vi "20220401.SA40289B 1D+2D in Air Dec.vi"() -> ()   [LabVIEW 2019]
uses:
  <userlib>/LevyLab/XY Utilities/subVIs/Get X and Y (multiple).vi
  <vilib>/Analysis/baseanly.llb/Mean (DBL).vi
  <userlib>/LevyLab/XY Utilities/subVIs/Linear Fit (single).vi
  <userlib>/LevyLab/XY Utilities/subVIs/Get X and Y (single).vi
  <userlib>/LevyLab/XY Utilities/Swap X and Y.vi
  <userlib>/LevyLab/XY Utilities/subVIs/Swap X and Y (single).vi
  <vilib>/Analysis/6fits.llb/Linear Fit Intervals.vi
  <vilib>/Analysis/6fits.llb/Confidence Interval (Linear).vi
  <userlib>/_OpenG.lib/file/file.llb/Build Path - Traditional__ogtk.vi
  <userlib>/LevyLab/XY Utilities/XY to 2D.vi
  <userlib>/LevyLab/Control VI/Other/Ramp_SubVI.vi
  <userlib>/LevyLab/LV-Data/LV-Data/LV-Data.lvclass
  <userlib>/LevyLab/XY Utilities/xy_utilities.lvlib
  <vilib>/Analysis/NI_AALBase.lvlib
panel:
  out "E_a":dbl[](array[numeric])
  out "Increasing Temp?":bool=TRUE
  out "Environment":enum16{"Air/Helium", "Vacuum"}(ring)
  in  "Tab Control":enum32{"Page 1", "Page 2"}(tab)
  out "G2T":cluster{dbl[], dbl[]}[](graph)
  out "Temp":cluster{dbl[], dbl[]}[](graph)
  out "Slopes vs Temp":cluster{dbl[], dbl[]}[](graph)
  out "Arrhenius":cluster{dbl[], dbl[]}[](graph)
  out "G4T 2D":cluster{dbl[], dbl[]}[](graph)
  out "G4T 1D":cluster{dbl[], dbl[]}[](graph)
  out "Temp 2":cluster{dbl[], dbl[]}[](graph)
  in  "Arrhenius?":bool=TRUE
  in  "2D Data?":bool=TRUE
  in  "Source Voltage":dbl=0.1
  in  "Init Temp":i32=275
  in  "Temp Step":i32=5
  in  "Final Temp":i32=300
  in  "Trimming":i32=400
  in  "Path":path=path "G:/.shortcut-targets-by-id/0B8-gGFa6hkR4XzJJMDlqZXVKRk0/ansom/Data/PPMS 2/SA40289B.20220401/00 - test/SA40289B.20220401.275K.dat"
  in  "One File?":bool
  in  "OK":bool
  in  "Update":bool
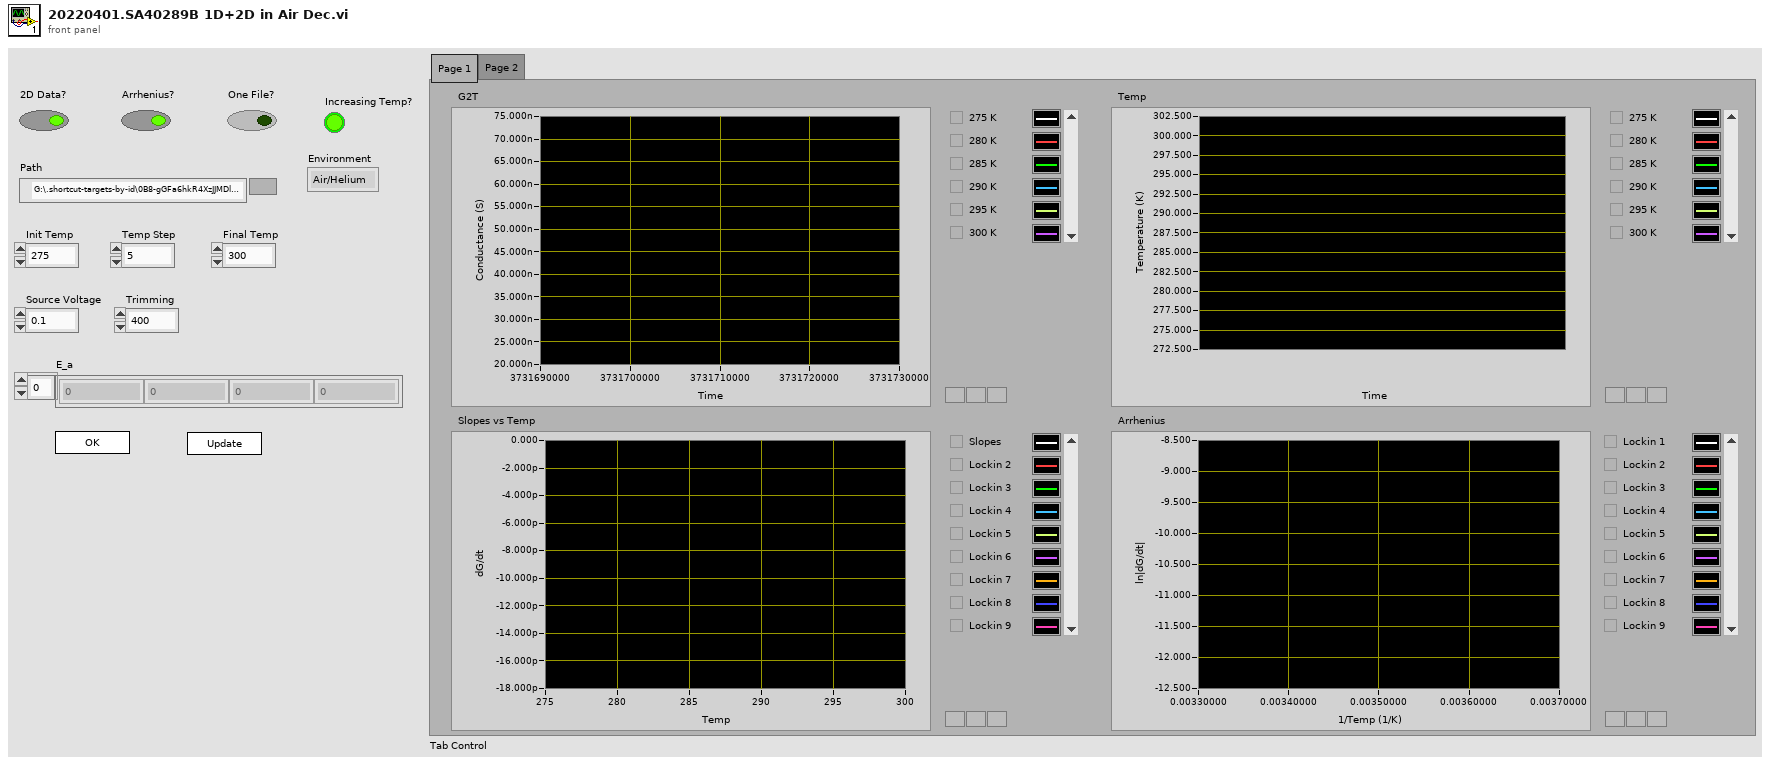
[diagram p1: front panel]
types:
  T1 = enum32{"Invalid", "Standard", "Closed", "Hidden", "Minimized", "Maximized"}
  T2 = enum32{"invalid app kind", "Development System", "Run Time System", "Student Edition", "Embedded LabVIEW", "Evaluation", "Custom"}
  T3 = cluster{"Core":cluster{"Current VI Reference":refnum<vi>, "Close Panel on Exit?":bool}, "G2T":cluster{dbl[], dbl[]}[], "G4T 1D":cluster{dbl[], dbl[]}[], "G4T 2D":cluster{dbl[], dbl[]}[], "Temp":cluster{dbl[], dbl[]}[], "Slopes":cluster{dbl[], dbl[]}[], "Source Voltage":dbl, "Final Temp":i32, "Init Temp":i32, "Temp Step":i32, "Trimming":i32, "Path":path, "One File?":bool}
  T4 = cluster{"Current VI Reference":refnum<vi>, "Close Panel on Exit?":bool}
  T5 = typedef "LV-Data.lvclass/Dictionary--cluster.ctl" = cluster{"key":string, "value":variant}
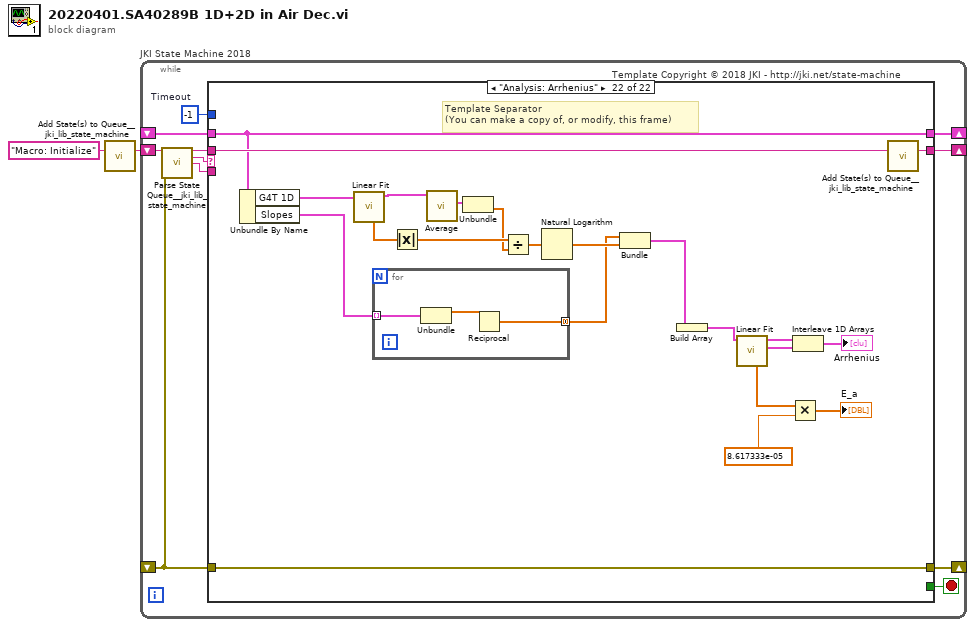
[diagram p0: block diagram]
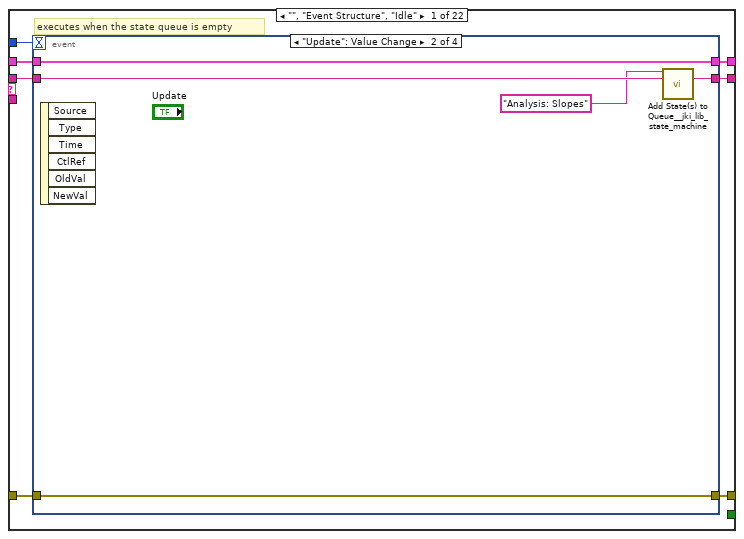
[diagram p2: hidden frame]
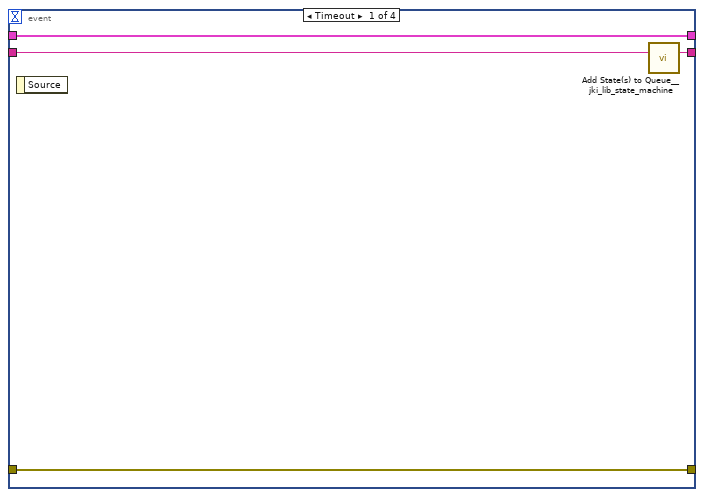
[diagram p3: hidden frame]
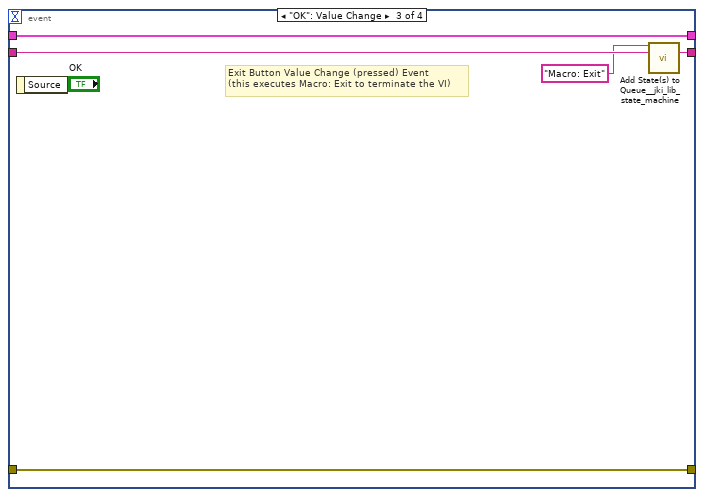
[diagram p4: hidden frame]
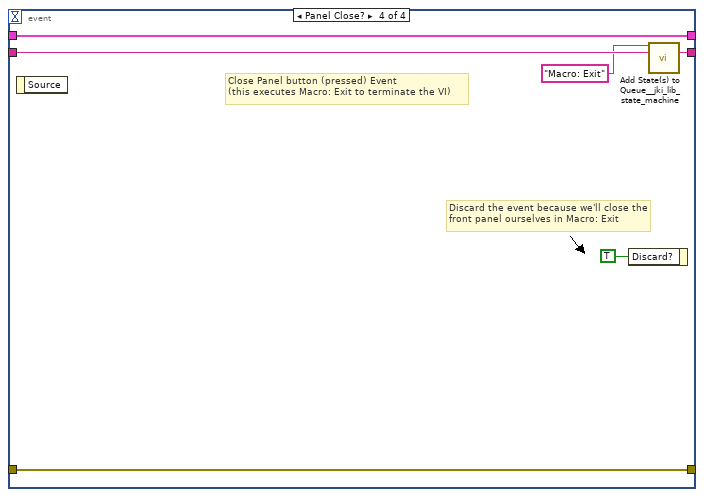
[diagram p5: hidden frame]
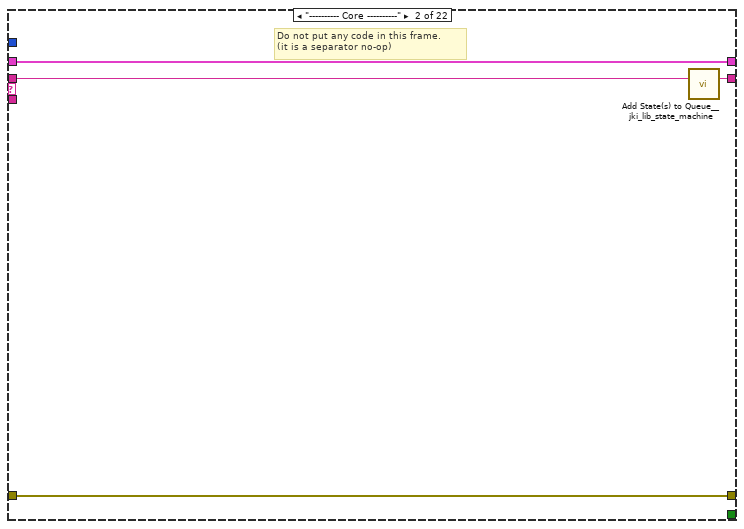
[diagram p6: hidden frame]
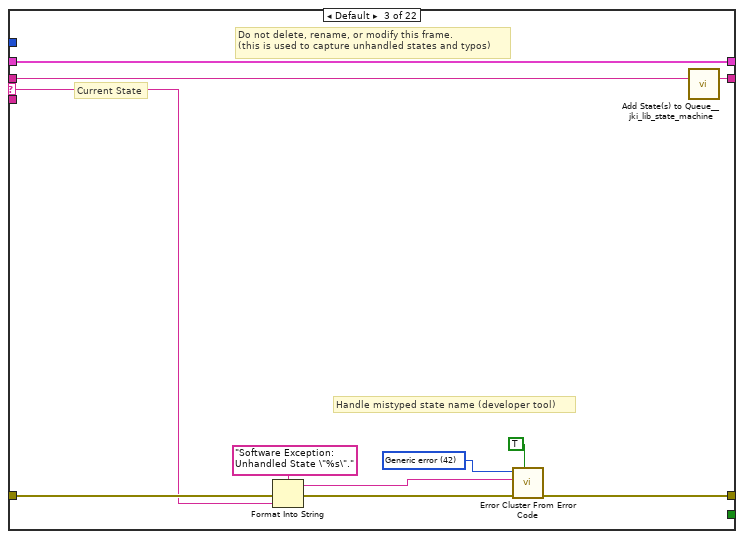
[diagram p7: hidden frame]
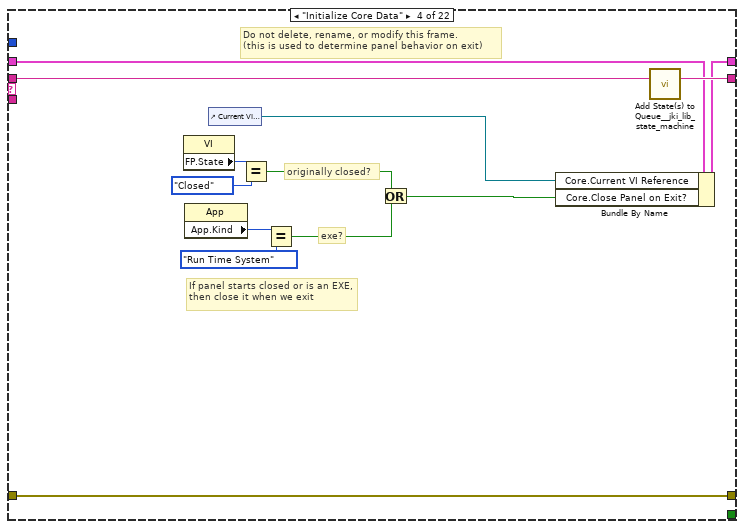
[diagram p8: hidden frame]
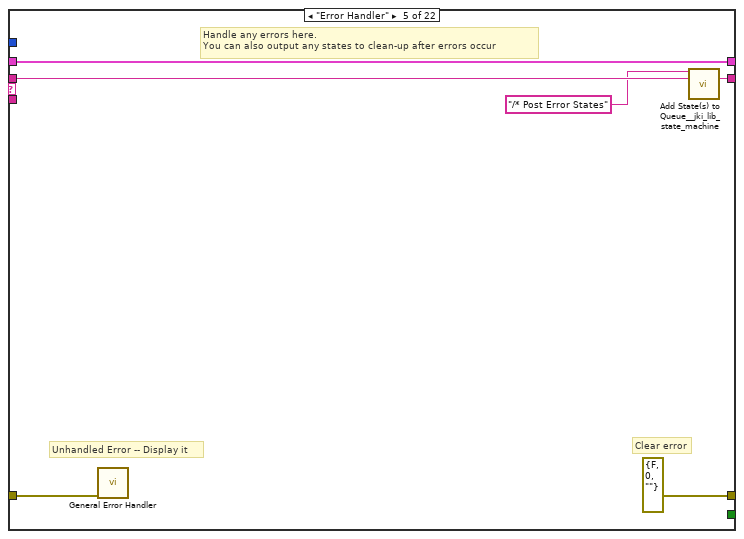
[diagram p9: hidden frame]
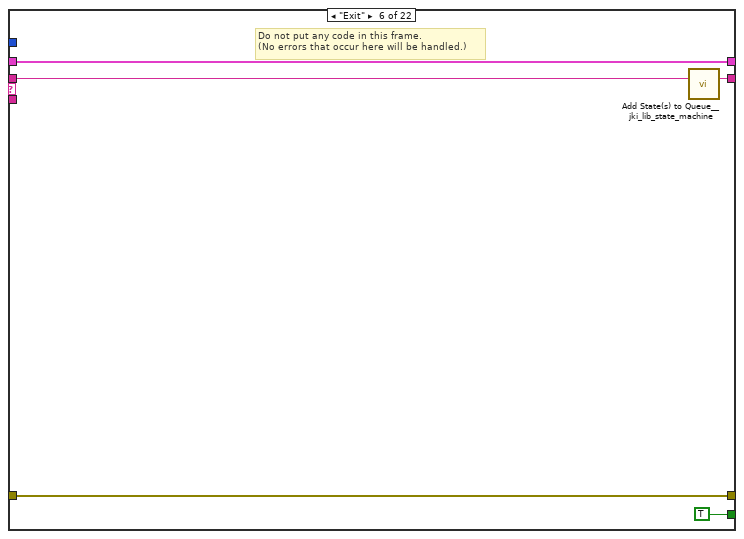
[diagram p10: hidden frame]
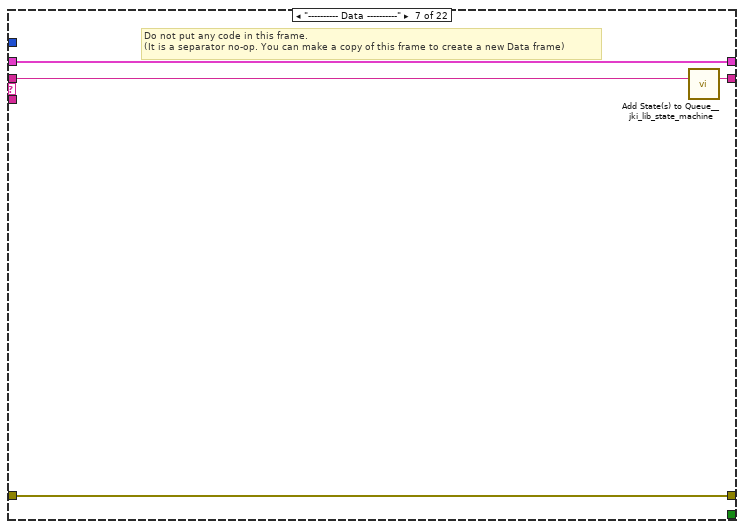
[diagram p11: hidden frame]
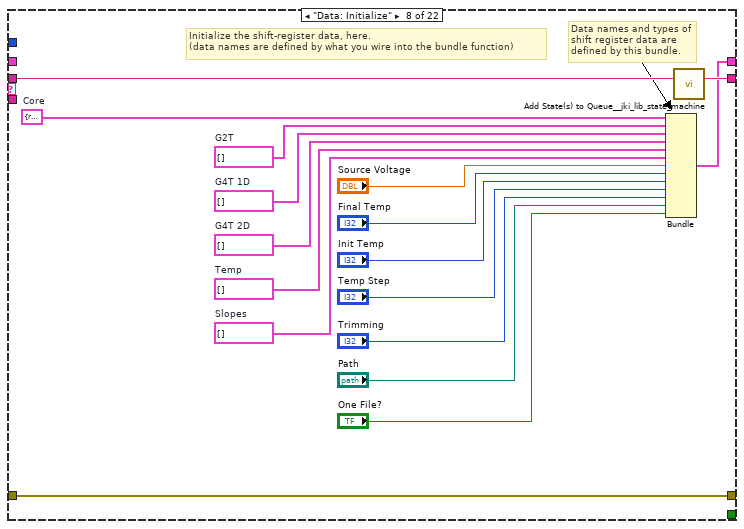
[diagram p12: hidden frame]
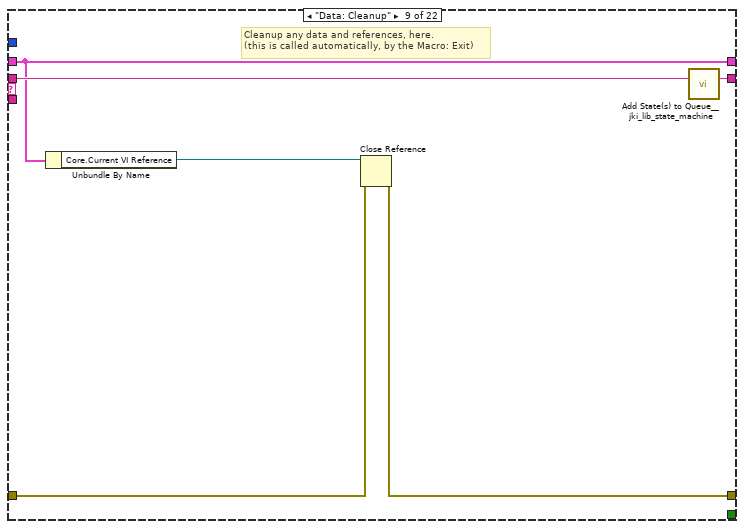
[diagram p13: hidden frame]
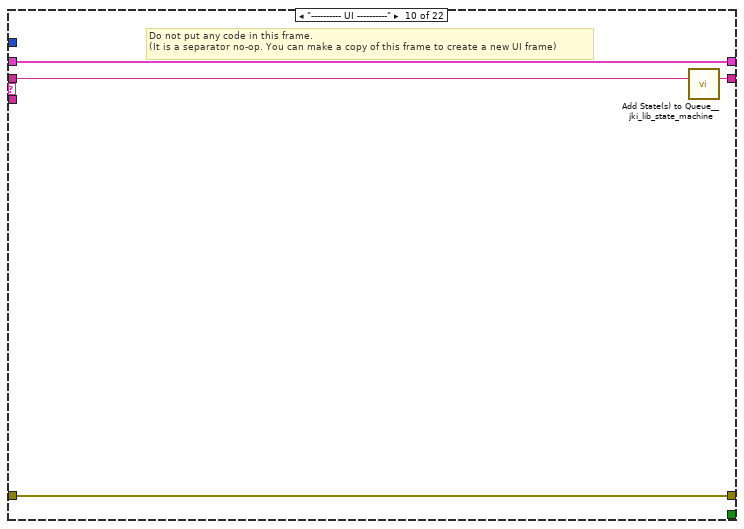
[diagram p14: hidden frame]
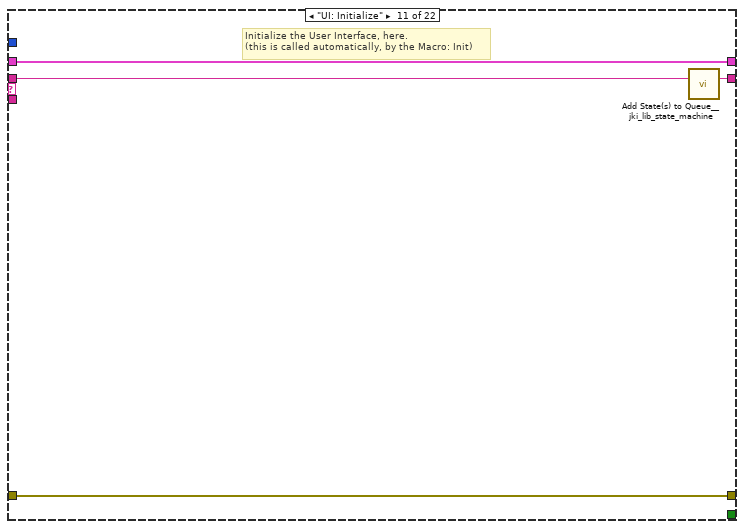
[diagram p15: hidden frame]
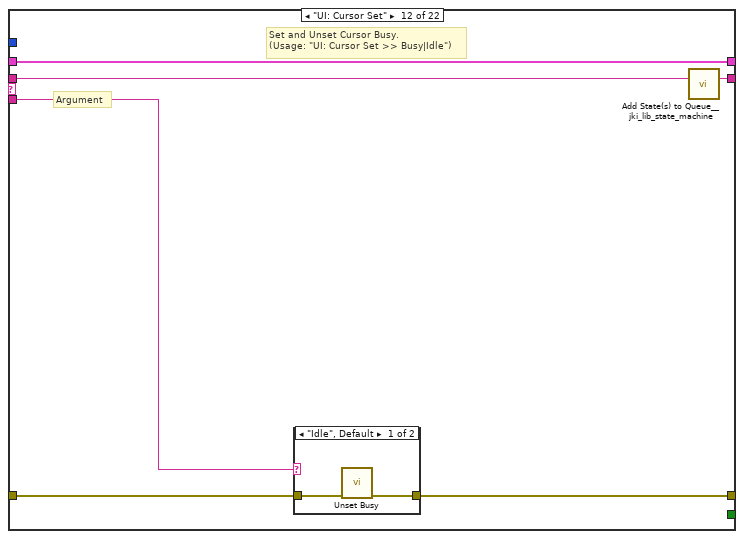
[diagram p16: hidden frame]
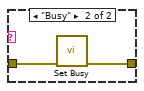
[diagram p17: hidden frame]
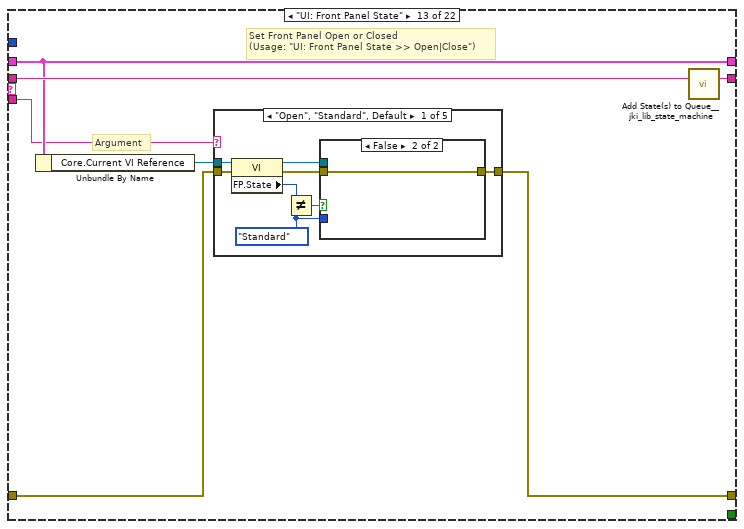
[diagram p18: hidden frame]
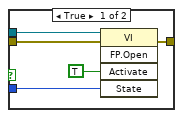
[diagram p19: hidden frame]
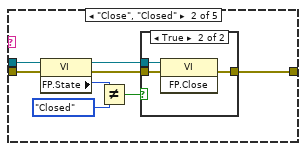
[diagram p20: hidden frame]
diagram:
  n1 = call <vilib>:"Add State(s) to Queue__jki_lib_state_machine.vi"("State(s) in (\"\")"="Macro: Initialize") -> ("States Out"=w2:string)  [unwired: 14 in]
  n2 = while "JKI State Machine 2018" {
    shift-right: [w6] -> _
    shift-left: _ -> [w3]
    shift-right: [w9] -> _
    shift-left: _ -> [w4]
    shift-right: [w8] -> _
    shift-left: w2 -> [w10]
    stop <- w7 stop-if-true
    w5 = -1  # Timeout
    # "Template Copyright © 2018 JKI - http://jki.net/state-machine"
    n3 = call <vilib>:"Parse State Queue__jki_lib_state_machine.vi"("State Queue"=w10, "Error In (no error)"=w4) -> ("Remaining States"=w12:string, "Current State"=w13:string, "Arguments"=w11:string)  [unwired: 11 in]
    n4 = case shown="\"Analysis: Arrhenius\"" w13 {
      selector: w13 -> [_ _ w45 _ _ _ _ _ _ _ _ _ _ _ _ _ _ _ _ _ _ _]
      tunnel: w12 -> [w20 w44 w49 w68 w74 w79 w83 w100 w106 w110 w114 w120 w131 w200 w215 w225 w229 w246 w317 w369 w384 w406]
      tunnel: w11 -> [_ _ _ _ _ _ _ _ _ _ _ w115 w125 _ _ _ _ _ _ _ _ _]
      tunnel: [w17 w42 w51 w65 errorcluster {"status"=FALSE, "code"=0, "source"=""} ("error out") w76 w81 w97 w102 w108 w111 w116 w128 w198 w213 w223 w227 w244 w315 w367 w382 w404] -> w9
      tunnel: w4 -> [w16 w42 w50 w65 w70 w76 w81 w97 w103 w108 w111 w117 w129 w198 w213 w223 w227 w244 w315 w367 w382 w404]
      tunnel: [w19 w43 w48 w67 w73 w78 w82 w99 w105 w109 w113 w119 w130 w199 w214 w224 w228 w245 w316 w368 w383 w405] -> w8
      tunnel: [_ _ _ _ _ TRUE _ _ _ _ _ _ _ _ _ _ _ _ _ _ _ _] -> w7
      tunnel: [w15 w41 w47 w66 w71 w77 w80 w98 w101 w107 w112 w118 w127 w197 w212 w222 w226 w238 w305 w366 w381 w403] -> w6
      tunnel: w5 -> [w14 _ _ _ _ _ _ _ _ _ _ _ _ _ _ _ _ _ _ _ _ _]
      tunnel: w3 -> [w18 w41 w47 w61 w71 w77 w80 _ w101 w107 w112 w118 w127 w197 w212 w222 w226 w239 w306 w365 w381 w403]
      frame "", "Event Structure", "Idle" {
        # "executes when the state queue is empty"
        n5 = event shown="[1] \"Update\": Value Change" {
          selector: _ -> [_ _ _ _]
          dyn-events: _ -> [_ _ _ _]
          timeout: w14 -> [_ _ _ _]
          tunnel: w20 -> [w24 w28 w34 w40]
          tunnel: [w23 w29 w33 w39] -> w19
          tunnel: w18 -> [w21 w27 w31 w37]
          tunnel: [w22 w25 w32 w38] -> w17
          tunnel: w16 -> [w22 w25 w32 w38]
          tunnel: [w21 w27 w31 w37] -> w15
          event Timeout {
            n6 = event-data() -> ()  [unwired: 1 in, 1 out]
            n7 = call <vilib>:"Add State(s) to Queue__jki_lib_state_machine.vi"("State(s) in (\"\")"=w24) -> ("States Out"=w23:string)  [unwired: 14 in]
          }
          event "Update": Value Change {
            n8 = event-data() -> ()  [unwired: 1 in, 6 out]
            n9 = call <vilib>:"Add State(s) to Queue__jki_lib_state_machine.vi"("State(s) in Front (\"\")"="Analysis: Slopes", "State(s) in (\"\")"=w28) -> ("States Out"=w29:string)  [unwired: 13 in]
          }
          event "OK": Value Change {
            # "Exit Button Value Change (pressed) Event\n(this executes Macro: Exit to terminate the VI)"
            n10 = event-data() -> ()  [unwired: 1 in, 1 out]
            n11 = call <vilib>:"Add State(s) to Queue__jki_lib_state_machine.vi"("State(s) in Front (\"\")"="Macro: Exit", "State(s) in (\"\")"=w34) -> ("States Out"=w33:string)  [unwired: 13 in]
          }
          event Panel Close? {
            # "Discard the event because we'll close the front panel ourselves in Macro: Exit"
            # "Close Panel button (pressed) Event\n(this executes Macro: Exit to terminate the VI)"
            n12 = event-data() -> ()  [unwired: 1 in, 1 out]
            n13 = event-data("Discard?"=TRUE) -> ()  [unwired: 1 in, 1 out]
            n14 = call <vilib>:"Add State(s) to Queue__jki_lib_state_machine.vi"("State(s) in Front (\"\")"="Macro: Exit", "State(s) in (\"\")"=w40) -> ("States Out"=w39:string)  [unwired: 13 in]
          }
        }
      }
      frame "---------- Core ----------" {
        # "Do not put any code in this frame.\n(it is a separator no-op)"
        n15 = call <vilib>:"Add State(s) to Queue__jki_lib_state_machine.vi"("State(s) in (\"\")"=w44) -> ("States Out"=w43:string)  [unwired: 14 in]
      }
      frame Default {
        w54 = 42 items=["No error", "Argument error", "Memory is full", "Out of zone", "End of file", "File already open", "Generic file I/O error", "File not found", "File permission error", "Disk is full", "Duplicate path", "Too many files open", "System feature not enabled", "Resource file not found", "Cannot add resource", "Resource not found", "Image not found", "Image memory error", "Pen does not exist", "Config type invalid", "Config token not found", "Config parse error", "Config memory error", "Bad external code format", "Bad external code offset", "External code not present", "Null window", "Destroy window error", "Null menu", "Print aborted", "Bad print record", "Print driver error", "Windows error during printing", "Memory error during printing", "Print dialog error", "Generic print error", "Invalid device refnum", "Device not found", "Device parameter error", "Device unit error", "Cannot open device", "Device call aborted", "Generic error", "Cancelled by user", "Object ID too low", "Object ID too high", "Object not in heap", "Unknown heap", "Unknown object (invalid DefProc)", "Unknown object (DefProc not in table)", "Message out of range", "Invalid (null) method", "Unknown message", "Manager call not supported", "Bad address", "Network operation in progress", "Network operation timed out", "Connection is busy", "Network attribute not supported", "Network error", "Address in use", "System out of memory", "Connection aborted", "Connection refused", "Not connected", "Already connected", "Connection closed", "Initialization error (interapplication manager)", "Bad occurrence", "Wait on unbound occurrence handler", "Occurrence queue overflow", "Datalog type conflict", "Unused", "Unrecognized type (interapplication manager)", "Memory corrupt", "Failed to make temporary DLL", "Old CIN version", "Drag socket not found", "Failed to load drop-object", "Failed to register OLE object", "Failed to release OLE object", "Format specifier type mismatch", "Unknown format specifier", "Too few format specifiers", "Too many format specifiers", "Scan failed", "Newer CIN version", "Error converting to variant", "Runtime menu error", "Password tampered", "Variant attribute not found", "Incompatible variant data type", "Event data is not available", "Event Store is not present", "Occurrence is not found", "Event Queue is not created", "Event info is not available", "Refnum passed is NULL", "Error retrieving Class GUID", "Error retrieving CoClass GUID", "Error retrieving TypeLib GUID.", "Bad built application magic bytes.", "Specific driver is different from the specific driver associated with the Logical Name.", "There is no session opened to the class driver.", "Max Error", "MAX - Error with config objects", "MAX - Error loading configuration", "MAX - Group not supported"]
        # "Current State"
        # "Do not delete, rename, or modify this frame.\n(this is used to capture unhandled states and typos)"
        # "Handle mistyped state name (developer tool)"
        n16 = Format Into String(format string="Software Exception: Unhandled State \"%s\"." ("message"), error in=w50, w45) -> (resulting string=w53:string, error out=w52:errorcluster)  [unwired: 1 in]
        n17 = call <vilib>:"Error Cluster From Error Code.vi"("show call chain? (False)"=TRUE, "error in (no error)"=w52, "error message (\"\")"=w53, "error code (0)"=w54) -> ("error out"=w51:errorcluster)  [unwired: 5 in]
        n18 = call <vilib>:"Add State(s) to Queue__jki_lib_state_machine.vi"("State(s) in (\"\")"=w49) -> ("States Out"=w48:string)  [unwired: 14 in]
      }
      frame "Initialize Core Data" {
        # "Do not delete, rename, or modify this frame.\n(this is used to determine panel behavior on exit)"
        # "originally closed?"
        # "exe?"
        # "If panel starts closed or is an EXE, then close it when we exit"
        n19 = property class="VI"() -> ("FP.State"=w58:T1)  [unwired: 2 in, 2 out]
        n20 = property class="App"() -> ("App.Kind"=w64:T2)  [unwired: 2 in, 2 out]
        n21 = control-ref of="Current VI Reference"() -> (w59:refnum<vi>)
        n22 = Equal?(x=w58, y=T1."Closed" ("Front Panel Window:State")) -> (x = y?=w56:bool)
        n23 = Equal?(x=w64, y=T2."Run Time System" ("Application:Kind")) -> (x = y?=w62:bool)
        n24 = Or(x=w56, y=w62) -> (x .or. y?=w60:bool)
        n25 = Bundle By Name(cluster=w61, "Core.Current VI Reference"=w59, "Core.Close Panel on Exit?"=w60) -> (w66:T3)
        n26 = call <vilib>:"Add State(s) to Queue__jki_lib_state_machine.vi"("State(s) in (\"\")"=w68) -> ("States Out"=w67:string)  [unwired: 14 in]
      }
      frame "Error Handler" {
        # "Unhandled Error -- Display it"
        # "Handle any errors here.\nYou can also output any states to clean-up after errors occur"
        # "Clear error"
        n27 = call <vilib>:"General Error Handler.vi"("error in (no error)"=w70) -> ()  [unwired: 10 in, 5 out]
        n28 = call <vilib>:"Add State(s) to Queue__jki_lib_state_machine.vi"("State(s) in Front (\"\")"="/* Post Error States", "State(s) in (\"\")"=w74) -> ("States Out"=w73:string)  [unwired: 13 in]
      }
      frame "Exit" {
        # "Do not put any code in this frame.\n(No errors that occur here will be handled.)"
        n29 = call <vilib>:"Add State(s) to Queue__jki_lib_state_machine.vi"("State(s) in (\"\")"=w79) -> ("States Out"=w78:string)  [unwired: 14 in]
      }
      frame "---------- Data ----------" {
        # "Do not put any code in this frame.\n(It is a separator no-op. You can make a copy of this frame to create a new Data frame)"
        n30 = call <vilib>:"Add State(s) to Queue__jki_lib_state_machine.vi"("State(s) in (\"\")"=w83) -> ("States Out"=w82:string)  [unwired: 14 in]
      }
      frame "Data: Initialize" {
        w91 = cluster{dbl[], dbl[]}[] []  # Slopes
        w92 = cluster{dbl[], dbl[]}[] []  # Temp
        w93 = cluster{dbl[], dbl[]}[] []  # G4T 2D
        w94 = cluster{dbl[], dbl[]}[] []  # G4T 1D
        w95 = cluster{dbl[], dbl[]}[] []  # G2T
        w96 = T4 {"Current VI Reference"=refnum, "Close Panel on Exit?"=FALSE}  # Core
        # "Data names and types of shift register data are defined by this bundle."
        # "Initialize the shift-register data, here.\n(data names are defined by what you wire into the bundle function)"
        n31 = Bundle("Core"=w96, "G2T"=w95, "G4T 1D"=w94, "G4T 2D"=w93, "Temp"=w92, "Slopes"=w91, "Source Voltage"="Source Voltage", "Final Temp"="Final Temp", "Init Temp"="Init Temp", "Temp Step"="Temp Step", "Trimming"="Trimming", "Path"="Path", "One File?"="One File?") -> (w98:T3)  [unwired: 1 in]
        n32 = call <vilib>:"Add State(s) to Queue__jki_lib_state_machine.vi"("State(s) in (\"\")"=w100) -> ("States Out"=w99:string)  [unwired: 14 in]
      }
      frame "Data: Cleanup" {
        # "Cleanup any data and references, here.\n(this is called automatically, by the Macro: Exit)"
        n33 = Unbundle By Name(w101) -> ("Core.Current VI Reference"=w104:refnum<vi>)
        n34 = Close Reference(reference=w104, error in (no error)=w103) -> (error out=w102:errorcluster)
        n35 = call <vilib>:"Add State(s) to Queue__jki_lib_state_machine.vi"("State(s) in (\"\")"=w106) -> ("States Out"=w105:string)  [unwired: 14 in]
      }
      frame "---------- UI ----------" {
        # "Do not put any code in this frame.\n(It is a separator no-op. You can make a copy of this frame to create a new UI frame)"
        n36 = call <vilib>:"Add State(s) to Queue__jki_lib_state_machine.vi"("State(s) in (\"\")"=w110) -> ("States Out"=w109:string)  [unwired: 14 in]
      }
      frame "UI: Initialize" {
        # "Initialize the User Interface, here.\n(this is called automatically, by the Macro: Init)"
        n37 = call <vilib>:"Add State(s) to Queue__jki_lib_state_machine.vi"("State(s) in (\"\")"=w114) -> ("States Out"=w113:string)  [unwired: 14 in]
      }
      frame "UI: Cursor Set" {
        # "Argument"
        # "Set and Unset Cursor Busy.\n(Usage: \"UI: Cursor Set >> Busy|Idle\")"
        n38 = case shown="\"Idle\", Default" w115 {
          tunnel: w117 -> [w122 w124]
          tunnel: [w121 w123] -> w116
          frame "Idle", Default {
            n39 = call <vilib>:"Unset Busy.vi"("error in (no error)"=w122) -> ("error out"=w121:errorcluster)  [unwired: 10 in]
          }
          frame "Busy" {
            n40 = call <vilib>:"Set Busy.vi"("error in (no error)"=w124) -> ("error out"=w123:errorcluster)  [unwired: 9 in, 1 out]
          }
        }
        n41 = call <vilib>:"Add State(s) to Queue__jki_lib_state_machine.vi"("State(s) in (\"\")"=w120) -> ("States Out"=w119:string)  [unwired: 14 in]
      }
      frame "UI: Front Panel State" {
        # "Argument"
        # "Set Front Panel Open or Closed\n(Usage: \"UI: Front Panel State >> Open|Close\")"
        n42 = Unbundle By Name(w127) -> ("Core.Current VI Reference"=w126:refnum<vi>)
        n43 = case shown="\"Open\", \"Standard\", Default" w125 {
          tunnel: w129 -> [w137 w152 w163 w176 w189]
          tunnel: [w139 w153 w165 w178 w191] -> w128
          tunnel: w126 -> [w138 w150 w164 w177 w190]
          frame "Open", "Standard", Default {
            w132 = T1."Standard" ("State")
            n44 = property class="VI"(reference=w138, error in=w137) -> (reference out=w135:refnum<vi>, error out=w136:errorcluster, "FP.State"=w134:T1)
            n45 = Not Equal?(x=w134, y=w132) -> (x != y?=w133:bool)
            n46 = case shown="False" w133 {
              tunnel: [w143 w145] -> w139
              tunnel: w136 -> [w142 w145]
              tunnel: w135 -> [w141 _]
              tunnel: w132 -> [w140 _]
              frame True {
                n47 = invoke class="VI" method="FP.Open"(reference=w141, error in=w142, "Activate"=TRUE, "State"=w140) -> (error out=w143:errorcluster)  [unwired: 1 in, 4 out]
              }
              frame False {
              }
            }
          }
          frame "Close", "Closed" {
            n48 = property class="VI"(reference=w150, error in=w152) -> (reference out=w149:refnum<vi>, error out=w151:errorcluster, "FP.State"=w147:T1)
            n49 = Not Equal?(x=w147, y=T1."Closed" ("Front Panel Window:State")) -> (x != y?=w146:bool)
            n50 = case shown="True" w146 {
              tunnel: [w154 w157] -> w153
              tunnel: w151 -> [w154 w156]
              tunnel: w149 -> [_ w155]
              frame False {
              }
              frame True {
                n51 = invoke class="VI" method="FP.Close"(reference=w155, error in=w156) -> (error out=w157:errorcluster)  [unwired: 1 in, 2 out]
              }
            }
          }
          frame "Hidden", "Hide" {
            w158 = T1."Hidden" ("State")
            n52 = property class="VI"(reference=w164, error in=w163) -> (reference out=w161:refnum<vi>, error out=w162:errorcluster, "FP.State"=w160:T1)
            n53 = Not Equal?(x=w160, y=w158) -> (x != y?=w159:bool)
            n54 = case shown="True" w159 {
              tunnel: [w169 w170] -> w165
              tunnel: w162 -> [w168 w170]
              tunnel: w161 -> [w167 _]
              tunnel: w158 -> [w166 _]
              frame True {
                n55 = invoke class="VI" method="FP.Open"(reference=w167, error in=w168, "State"=w166) -> (error out=w169:errorcluster)  [unwired: 2 in, 4 out]
              }
              frame False {
              }
            }
          }
          frame "Minimize", "Minimized" {
            w171 = T1."Minimized" ("State")
            n56 = property class="VI"(reference=w177, error in=w176) -> (reference out=w174:refnum<vi>, error out=w175:errorcluster, "FP.State"=w173:T1)
            n57 = Not Equal?(x=w173, y=w171) -> (x != y?=w172:bool)
            n58 = case shown="True" w172 {
              tunnel: [w182 w183] -> w178
              tunnel: w175 -> [w181 w183]
              tunnel: w174 -> [w180 _]
              tunnel: w171 -> [w179 _]
              frame True {
                n59 = invoke class="VI" method="FP.Open"(reference=w180, error in=w181, "State"=w179) -> (error out=w182:errorcluster)  [unwired: 2 in, 4 out]
              }
              frame False {
              }
            }
          }
          frame "Maximize", "Maximized" {
            w184 = T1."Maximized" ("State")
            n60 = property class="VI"(reference=w190, error in=w189) -> (reference out=w187:refnum<vi>, error out=w188:errorcluster, "FP.State"=w186:T1)
            n61 = Not Equal?(x=w186, y=w184) -> (x != y?=w185:bool)
            n62 = case shown="True" w185 {
              tunnel: [w195 w196] -> w191
              tunnel: w188 -> [w194 w196]
              tunnel: w187 -> [w193 _]
              tunnel: w184 -> [w192 _]
              frame True {
                n63 = invoke class="VI" method="FP.Open"(reference=w193, error in=w194, "State"=w192) -> (error out=w195:errorcluster)  [unwired: 2 in, 4 out]
              }
              frame False {
              }
            }
          }
        }
        n64 = call <vilib>:"Add State(s) to Queue__jki_lib_state_machine.vi"("State(s) in (\"\")"=w131) -> ("States Out"=w130:string)  [unwired: 14 in]
      }
      frame "---------- Macro ----------" {
        # "Do not put any code in this frame.\n(It is a separator no-op. You can make a copy of this frame to create a new Macro frame)"
        n65 = call <vilib>:"Add State(s) to Queue__jki_lib_state_machine.vi"("State(s) in (\"\")"=w200) -> ("States Out"=w199:string)  [unwired: 14 in]
      }
      frame "Macro: Initialize" {
        w205 = ""
        # "Initialization Macro\n(This is called once, when the VI starts)"
        n66 = Select(t="Analysis: Arrhenius", s="Arrhenius?", f=w205) -> (s? t:f=w203:string)
        n67 = Select(t="Analysis: 2D Data\nAnalysis: Slopes", s="2D Data?", f=w205) -> (s? t:f=w204:string)
        n68 = call <vilib>:"Add State(s) to Queue__jki_lib_state_machine.vi"("State(s) in Front (\"\")"=w204, "State(s) in (\"\")"=w203, "State(s) at Back (\"\")"="Analysis: Plot G vs t") -> ("States Out"=w201:string)  [unwired: 12 in]
        n69 = call <vilib>:"Add State(s) to Queue__jki_lib_state_machine.vi"("State(s) in Front (\"\")"="Data: Initialize\nInitialize Core Data\nUI: Initialize\nUI: Front Panel State >> Open\nAnalysis: Load 1D\nAnalysis: Slopes", "State(s) in (\"\")"=w201) -> ("States Out"=w210:string)  [unwired: 13 in]
        n70 = call <vilib>:"Add State(s) to Queue__jki_lib_state_machine.vi"("State(s) in Front (\"\")"=w210, "State(s) in (\"\")"=w215) -> ("States Out"=w214:string)  [unwired: 13 in]
      }
      frame "Macro: Exit" {
        # "Exit Macro\n(This is called once, when the VI exits)"
        n71 = Unbundle By Name(w222) -> ("Core.Close Panel on Exit?"=w221:bool)
        n72 = Select(t="UI: Front Panel State >> Close", s=w221, f="") -> (s? t:f=w218:string)
        n73 = call <vilib>:"Add State(s) to Queue__jki_lib_state_machine.vi"("State(s) in (\"\")"=w218, "State(s) at Back (\"\")"="Data: Cleanup\nExit") -> ("States Out"=w216:string)  [unwired: 13 in]
        n74 = call <vilib>:"Add State(s) to Queue__jki_lib_state_machine.vi"("State(s) in Front (\"\")"=w216, "State(s) in (\"\")"=w225) -> ("States Out"=w224:string)  [unwired: 13 in]
      }
      frame "---------- Analysis ----------" {
        # "Template Separator\n(You can make a copy of, or modify, this frame)"
        n75 = call <vilib>:"Add State(s) to Queue__jki_lib_state_machine.vi"("State(s) in (\"\")"=w229) -> ("States Out"=w228:string)  [unwired: 14 in]
      }
      frame "Analysis: Load 1D" {
        n76 = Unbundle By Name(w239) -> ("Source Voltage"=w240:dbl, "Final Temp"=w235:i32, "Init Temp"=w233:i32, "Temp Step"=w232:i32, "Path"=w242:path, "Trimming"=w241:i32, "One File?"=w243:bool)
        n77 = Subtract(x=w235, y=w233) -> (x-y=w234:i32)
        n78 = Divide(x=w234, y=w232) -> (x/y=w231:dbl)
        n79 = Increment(x=w231) -> (x+1=w230:dbl)
        n80 = case shown="False" w243 {
          tunnel: w242 -> [w253 w302]
          tunnel: w241 -> [w250 w294]
          tunnel: w240 -> [w249 w293]
          tunnel: [w248 w285] -> w237
          tunnel: [w247 w284] -> w236
          tunnel: w233 -> [w252 _]
          tunnel: w232 -> [w251 _]
          tunnel: w230 -> [w254 _]
          frame False {
            n81 = for {
              N: w254 -> [_]
              tunnel: w253 -> [w278]
              tunnel: w252 -> [w281]
              tunnel: w251 -> [w282]
              tunnel: w250 -> [w265]
              tunnel: w249 -> [w260]
              tunnel: [w256] -> w248 mode=indexing
              tunnel: [w255] -> w247 mode=indexing
              i -> [w283]
              n82 = Multiply(x=w282, y=w283) -> (x*y=w280:i32)
              n83 = Strip Path(path=w278) -> (stripped path=w271:path, name=w277:string)
              n84 = Add(x=w281, y=w280) -> (x+y=w279:i32)
              n85 = Format Into String(w279) -> (resulting string=w275:string)  [unwired: 3 in, 1 out]
              n86 = String Subset(string=w277, length (rest)=18) -> (substring=w273:string)  [unwired: 1 in]
              n87 = Concatenate Strings(w273, w275, "K.dat") -> (w272:string)
              n88 = call-poly <userlib>:"Build Path__ogtk.vi"("name or relative path"=w272, "base path"=w271) -> ("appended path"=w270:path)
              n89 = call <userlib>:"Data Read.vi"("path"=w270) -> ("Data (Dictionary)"=w269:T5[])  [unwired: 7 in, 3 out]
              n90 = call "Read Dictionary.vi"("Numeric"=0, "Dictionary In"=w269) -> ("data"=w264:dbl[])
              n91 = call "Read Dictionary.vi"("Numeric"=4, "Dictionary In"=w269) -> ("data"=w263:dbl[])
              n92 = call "Read Dictionary.vi"("Numeric"=1, "Dictionary In"=w269) -> ("data"=w262:dbl[])
              n93 = Array Subset(array=w264, index=w265) -> (w259:dbl[])  [unwired: 1 in]
              n94 = Array Subset(array=w263, index=w265) -> (w261:dbl[])  [unwired: 1 in]
              n95 = Array Subset(array=w262, index=w265) -> (w258:dbl[])  [unwired: 1 in]
              n96 = Divide(x=w261, y=w260) -> (x/y=w257:dbl[])
              n97 = Bundle(w259, w258) -> (w255:cluster{dbl[], dbl[]})  [unwired: 1 in]
              n98 = Bundle(w259, w257) -> (w256:cluster{dbl[], dbl[]})  [unwired: 1 in]
            }
          }
          frame True {
            n99 = call <userlib>:"Data Read.vi"("path"=w302) -> ("Data (Dictionary)"=w301:T5[])  [unwired: 7 in, 3 out]
            n100 = call "Read Dictionary.vi"("Numeric"=0, "Dictionary In"=w301) -> ("data"=w295:dbl[])
            n101 = call "Read Dictionary.vi"("Numeric"=5, "Dictionary In"=w301) -> ("data"=w296:dbl[])
            n102 = call "Read Dictionary.vi"("Numeric"=1, "Dictionary In"=w301) -> ("data"=w297:dbl[])
            n103 = Array Subset(array=w295, index=w294) -> (w286:dbl[])  [unwired: 1 in]
            n104 = Array Subset(array=w296, index=w294) -> (w292:dbl[])  [unwired: 1 in]
            n105 = Array Subset(array=w297, index=w294) -> (w287:dbl[])  [unwired: 1 in]
            n106 = Divide(x=w292, y=w293) -> (x/y=w291:dbl[])
            n107 = Absolute Value(x=w291) -> (abs(x)=w290:dbl[])
            n108 = Bundle(w286, w290) -> (w289:cluster{dbl[], dbl[]})  [unwired: 1 in]
            n109 = Bundle(w286, w287) -> (w288:cluster{dbl[], dbl[]})  [unwired: 1 in]
            n110 = Build Array(w289) -> (w285:cluster{dbl[], dbl[]}[])
            n111 = Build Array(w288) -> (w284:cluster{dbl[], dbl[]}[])
          }
        }
        n112 = call <vilib>:"Add State(s) to Queue__jki_lib_state_machine.vi"("State(s) in (\"\")"=w246) -> ("States Out"=w245:string)  [unwired: 14 in]
        n113 = Bundle By Name(cluster=w239, "G2T"=w237, "Temp"=w236) -> (w238:T3)
      }
      frame "Analysis: 2D Data" {
        # "Your code here.\n(You can make a copy of, or modify, this frame)"
        n114 = Unbundle By Name(w306) -> ("Final Temp"=w310:i32, "Init Temp"=w309:i32, "Temp Step"=w308:i32, "Path"=w314:path, "Trimming"=w313:i32)
        n115 = Subtract(x=w310, y=w309) -> (x-y=w312:i32)
        n116 = Divide(x=w312, y=w308) -> (x/y=w311:dbl)
        n117 = Increment(x=w311) -> (x+1=w307:dbl)
        n118 = for {
          N: w307 -> [_]
          tunnel: w314 -> [w353]
          tunnel: w308 -> [w356]
          tunnel: w313 -> [w327]
          tunnel: [w337] -> w304 mode=indexing
          tunnel: [w336] -> w303 mode=indexing
          tunnel: w309 -> [w335]
          i -> [w357]
          n119 = Multiply(x=w356, y=w357) -> (x*y=w355:i32)
          n120 = Strip Path(path=w353) -> (stripped path=w346:path, name=w352:string)
          n121 = Add(x=w335, y=w355) -> (x+y=w354:i32)
          n122 = Format Into String(w354) -> (resulting string=w350:string)  [unwired: 3 in, 1 out]
          n123 = String Subset(string=w352, length (rest)=18) -> (substring=w348:string)  [unwired: 1 in]
          n124 = Concatenate Strings(w348, w350, "K.dat") -> (w347:string)
          n125 = call-poly <userlib>:"Build Path__ogtk.vi"("name or relative path"=w347, "base path"=w346) -> ("appended path"=w345:path)
          n126 = call <userlib>:"Data Read.vi"("path"=w345) -> ("Data (Dictionary)"=w332:T5[])  [unwired: 7 in, 3 out]
          n127 = call "Read Dictionary.vi"("Numeric"=0, "Dictionary In"=w332) -> ("data"=w341:dbl[])
          n128 = call "Read Dictionary.vi"("Numeric"=4, "Dictionary In"=w332) -> ("data"=w329:dbl[])
          n129 = call "Read Dictionary.vi"("Numeric"=6, "Dictionary In"=w332) -> ("data"=w340:dbl[])
          n130 = call "Read Dictionary.vi"("Numeric"=5, "Dictionary In"=w332) -> ("data"=w328:dbl[])
          n131 = call "Read Dictionary.vi"("Numeric"=6, "Dictionary In"=w332) -> ("data"=w339:dbl[])
          n132 = call "Read Dictionary.vi"("Numeric"=10, "Dictionary In"=w332) -> ("data"=w330:dbl[])
          n133 = Array Subset(array=w341, index=w327) -> (w338:dbl[])  [unwired: 1 in]
          n134 = Array Subset(array=w329, index=w327) -> (w319:dbl[])  [unwired: 1 in]
          n135 = Array Subset(array=w340, index=w327) -> (w326:dbl[])  [unwired: 1 in]
          n136 = Array Subset(array=w328, index=w327) -> (w325:dbl[])  [unwired: 1 in]
          n137 = Array Subset(array=w339, index=w327) -> (w322:dbl[])  [unwired: 1 in]
          n138 = Array Subset(array=w330, index=w327) -> (w321:dbl[])  [unwired: 1 in]
          n139 = Subtract(x=w326, y=w325) -> (x-y=w324:dbl[])
          n140 = Subtract(x=w322, y=w321) -> (x-y=w318:dbl[])
          n141 = Divide(x=w319, y=w324) -> (x/y=w323:dbl[])
          n142 = Divide(x=w319, y=w318) -> (x/y=w320:dbl[])
          n143 = Bundle(w338, w320) -> (w336:cluster{dbl[], dbl[]})  [unwired: 1 in]
          n144 = Bundle(w338, w323) -> (w337:cluster{dbl[], dbl[]})  [unwired: 1 in]
        }
        n145 = call <vilib>:"Add State(s) to Queue__jki_lib_state_machine.vi"("State(s) in (\"\")"=w317) -> ("States Out"=w316:string)  [unwired: 14 in]
        n146 = Bundle By Name(cluster=w306, "G4T 1D"=w304, "G4T 2D"=w303) -> (w305:T3)
      }
      frame "Analysis: Slopes" {
        # "Template Separator\n(You can make a copy of, or modify, this frame)"
        n147 = Unbundle By Name(w365) -> ("Temp"=w362:cluster{dbl[], dbl[]}[], "G4T 2D"=w363:cluster{dbl[], dbl[]}[])
        n148 = call <userlib>:"Linear Fit (multiple).vi"("XY-data"=w363) -> ("slopes"=w359:dbl[])  [unwired: 4 in, 6 out]
        n149 = call-poly <userlib>:"Get X and Y.vi"("XY-data"=w362) -> ("Y-Arrays"=w361:cluster{"Y-array":dbl[]}[])  [unwired: 7 in, 3 out]
        n150 = for {
          tunnel: w361 -> [w373] mode=indexing
          tunnel: [w370] -> w360 mode=indexing
          n151 = Unbundle By Name(w373) -> ("Y-array"=w372:dbl[])
          n152 = call-poly <vilib>:"Mean.vi"("X"=w372) -> ("mean"=w371:dbl)  [unwired: 1 out]
          n153 = Round To Nearest(number=w371) -> (nearest integer value=w370:dbl)
        }
        n154 = Bundle(w360, "slopes"=w359) -> (w358:cluster{dbl[], "slopes":dbl[]})  [unwired: 1 in]
        n155 = Build Array(w358) -> (w364:cluster{dbl[], "slopes":dbl[]}[])
        n156 = call <vilib>:"Add State(s) to Queue__jki_lib_state_machine.vi"("State(s) in (\"\")"=w369) -> ("States Out"=w368:string)  [unwired: 14 in]
        n157 = Bundle By Name(cluster=w365, "Slopes"=w364) -> (w366:T3)
      }
      frame "Analysis: Plot G vs t" {
        # "Template Separator\n(You can make a copy of, or modify, this frame)"
        n158 = Unbundle By Name(w381) -> ("G2T"=→"G2T":cluster{dbl[], dbl[]}[], "G4T 1D"=→"G4T 1D":cluster{dbl[], dbl[]}[], "G4T 2D"=→"G4T 2D":cluster{dbl[], dbl[]}[], "Temp"=→"Temp" →"Temp 2":cluster{dbl[], dbl[]}[], "Slopes"=→"Slopes vs Temp":cluster{dbl[], dbl[]}[])
        n159 = call <vilib>:"Add State(s) to Queue__jki_lib_state_machine.vi"("State(s) in (\"\")"=w384) -> ("States Out"=w383:string)  [unwired: 14 in]
        "Increasing Temp?" <- FALSE
        "Environment" <- enum16{"Air/Helium", "Vacuum"}."Air/Helium" ("Environment")
      }
      frame "Analysis: Arrhenius" {
        # "Template Separator\n(You can make a copy of, or modify, this frame)"
        n160 = Unbundle By Name(w403) -> ("G4T 1D"=w402:cluster{dbl[], dbl[]}[], "Slopes"=w387:cluster{dbl[], dbl[]}[])
        n161 = call-poly <vilib>:"Linear Fit.vi"("XY-data"=w402) -> ("XY-data out"=w400:cluster{"X-array":dbl[], "Y-array":dbl[]}[], "slopes"=w401:dbl[])  [unwired: 4 in, 5 out]
        n162 = for {
          tunnel: w387 -> [w409] mode=indexing
          tunnel: [w408] -> w386 mode=concatenating
          n163 = Unbundle(w409) -> (w407:dbl[])  [unwired: 1 out]
          n164 = Reciprocal(x=w407) -> (1/x=w408:dbl[])
        }
        n165 = Absolute Value(x=w401) -> (abs(x)=w399:dbl[])
        n166 = call <userlib>:"Average.vi"("XY-data"=w400) -> ("Averaged XY-data out"=w398:cluster{"X-array":dbl[], "Y-array":dbl[]})  [unwired: 8 in, 2 out]
        n167 = Unbundle(w398) -> ("Y-array"=w397:dbl[])  [unwired: 1 out]
        n168 = Divide(x=w399, y=w397) -> (x/y=w396:dbl[])
        n169 = Natural Logarithm(1:w396) -> (0:w395:dbl[])
        n170 = Bundle(w386, w395) -> (w394:cluster{dbl[], dbl[]})  [unwired: 1 in]
        n171 = Build Array(w394) -> (w385:cluster{dbl[], dbl[]}[])
        n172 = call-poly <vilib>:"Linear Fit.vi"("XY-data"=w385) -> ("Best Fits"=w392:cluster{"X-array":dbl[], "Y-array":dbl[]}[], "XY-data out"=w393:cluster{"X-array":dbl[], "Y-array":dbl[]}[], "slopes"=w390:dbl[])  [unwired: 4 in, 4 out]
        n173 = Multiply(x=w390, y=8.617333e-05) -> (x*y=→"E_a":dbl[])
        n174 = Interleave 1D Arrays(w393, w392) -> (→"Arrhenius":cluster{"X-array":dbl[], "Y-array":dbl[]}[])
        n175 = call <vilib>:"Add State(s) to Queue__jki_lib_state_machine.vi"("State(s) in (\"\")"=w406) -> ("States Out"=w405:string)  [unwired: 14 in]
      }
    }
  }
